vi "indexArray_ex1.vi"() -> ()   [LabVIEW 2020]
panel:
  in  "disabled index (row) 2":i32
  out "subarray":i32[](array[numeric])
  out "Array":i32[][](array[numeric])
  out "appended array":dbl[](array[numeric])
  out "x+y":dbl
  in  "stop":bool
  in  "Numeric":dbl
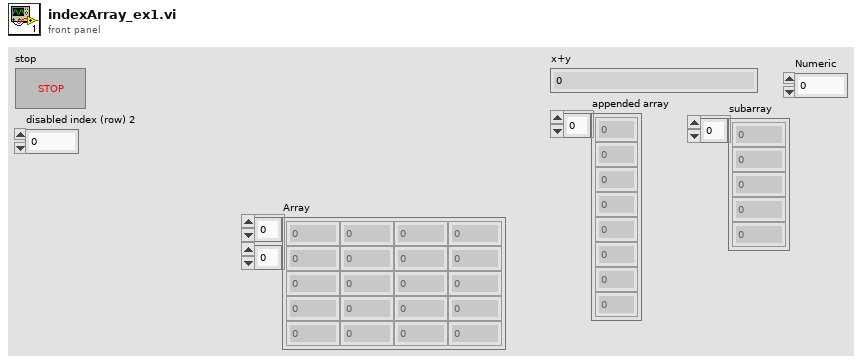
[diagram p1: front panel]
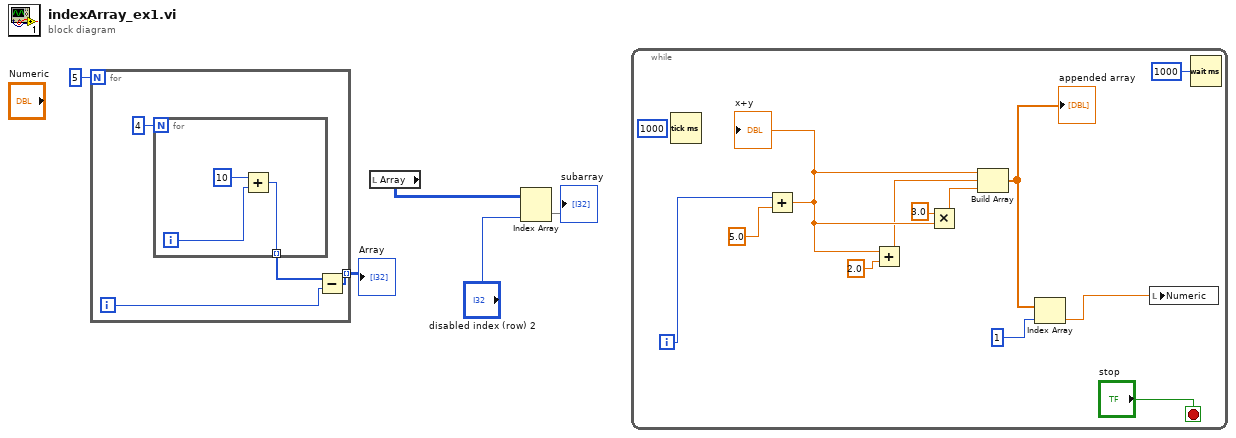
[diagram p0: block diagram]
diagram:
  n1 = for {
    N: 5 -> [_]
    tunnel: [w6] -> w4 mode=indexing
    i -> [w8]
    n2 = for {
      N: 4 -> [_]
      tunnel: [w10] -> w7 mode=indexing
      i -> [w12]
      n3 = Add(x=10, y=w12) -> (x+y=w10:i32)
    }
    n4 = Subtract(x=w7, y=w8) -> (x-y=w6:i32[])
  }
  "Array" <- w4
  n5 = local read "Array"() -> (w3:i32[][])
  n6 = Index Array(array=w3, index (col)="disabled index (row) 2") -> (element=→"subarray":i32[])  [unwired: 1 in]
  n7 = while {
    i -> [w23]
    stop <- "stop" stop-if-true
    (unwired) u32 1000 ("millisecond timer value")
    n8 = Tick Count (ms)() -> ()  [unwired: 1 out]
    n9 = Add(x=w23, y=5.0) -> (x+y=w17:dbl)
    "x+y" <- w17
    n10 = Add(x=w17, y=2.0) -> (x+y=w16:dbl)
    n11 = Multiply(x=3.0, y=w17) -> (x*y=w14:dbl)
    n12 = Build Array(w17, w16, w14) -> (w21:dbl[])
    "appended array" <- w21
    n13 = Index Array(array=w21, index=1) -> (element=w22:dbl)
    n14 = local write "Numeric"(w22) -> ()
    n15 = Wait (ms)(milliseconds to wait=u32 1000) -> ()  [unwired: 1 out]
  }
